vi "EFMC-3.vi"(11 "数组":u8[](array[numeric])) -> (0 "传感器信号":cluster{"陀螺温度":i16, "加计温度":i16}, 1 "组合数据来源字":T1, 2 "对准数据来源字":cluster{"位置数据":string, "姿态数据":string}, 3 "系统工作状态字":cluster{"工作状态":string, "工作模式":string})   [LabVIEW 2012]
uses:
  index-i16.vi
  XX-I16.vi
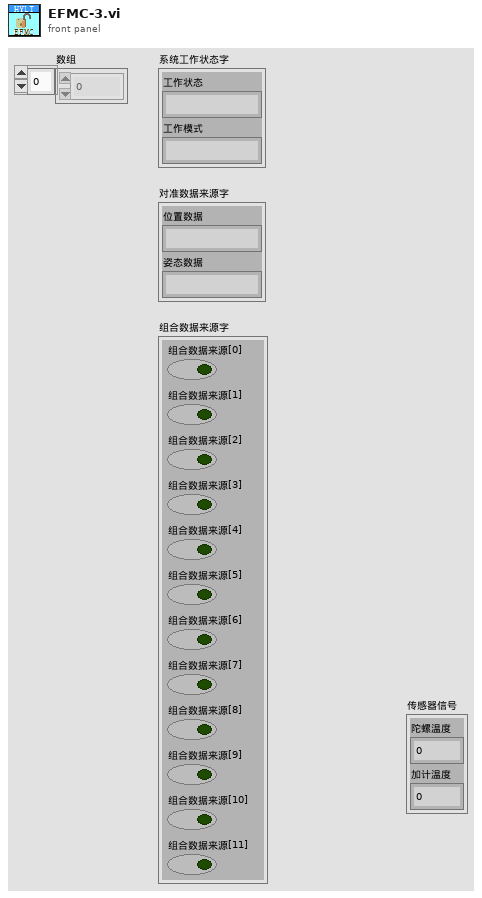
[diagram p1: front panel]
types:
  T1 = cluster{"组合数据来源[0]":bool, "组合数据来源[1]":bool, "组合数据来源[2]":bool, "组合数据来源[3]":bool, "组合数据来源[4]":bool, "组合数据来源[5]":bool, "组合数据来源[6]":bool, "组合数据来源[7]":bool, "组合数据来源[8]":bool, "组合数据来源[9]":bool, "组合数据来源[10]":bool, "组合数据来源[11]":bool}
  T2 = cluster{"GNSS1+GPS":bool, "GNSS1BD":bool, "GCSS1+GLO":bool, "GNSS3+GPS":bool, "GNSS2+GPS":bool, "GNSS2BD":bool, "GNSS2+GLO":bool, "GNSS3BD":bool, "GNSS3+GLO":bool, "大气数据":bool, "星敏1数据":bool, "星敏2数据":bool}
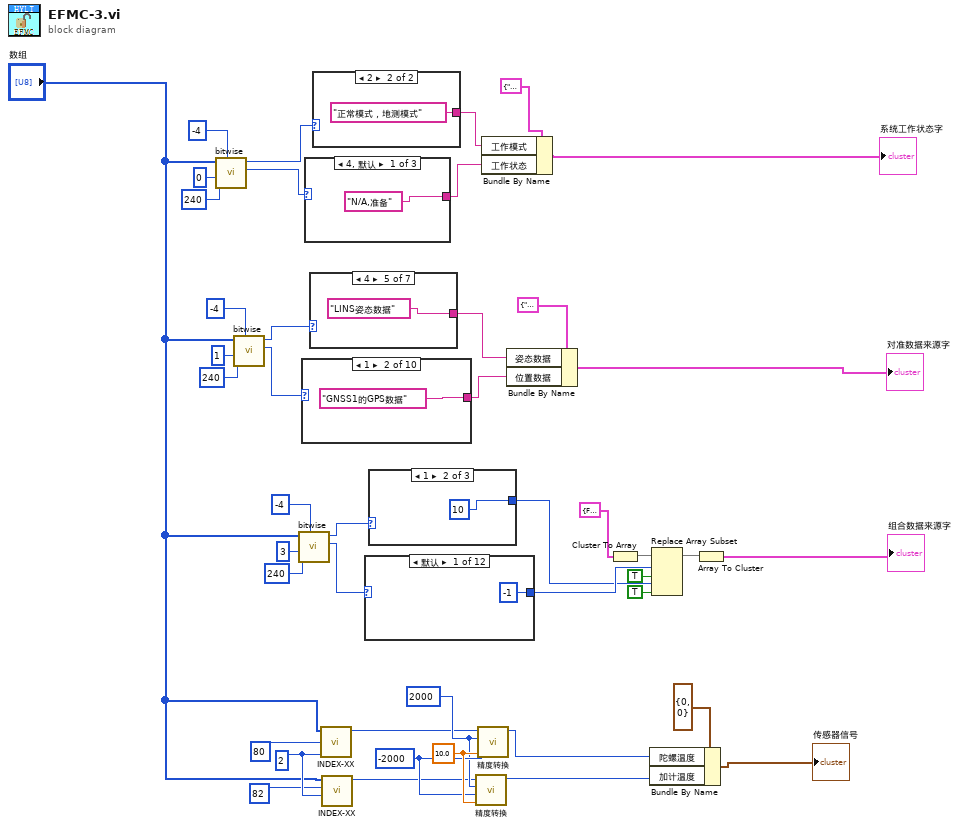
[diagram p0: block diagram]
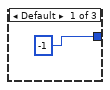
[diagram p2: hidden frame]
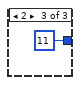
[diagram p3: hidden frame]
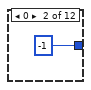
[diagram p4: hidden frame]
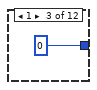
[diagram p5: hidden frame]
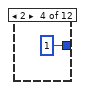
[diagram p6: hidden frame]
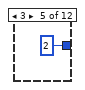
[diagram p7: hidden frame]
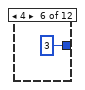
[diagram p8: hidden frame]
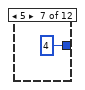
[diagram p9: hidden frame]
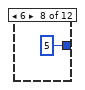
[diagram p10: hidden frame]
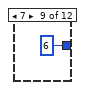
[diagram p11: hidden frame]
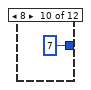
[diagram p12: hidden frame]
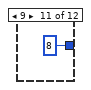
[diagram p13: hidden frame]
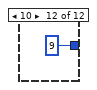
[diagram p14: hidden frame]
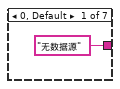
[diagram p15: hidden frame]
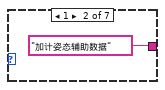
[diagram p16: hidden frame]
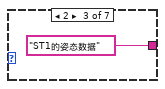
[diagram p17: hidden frame]
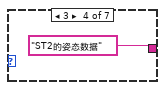
[diagram p18: hidden frame]
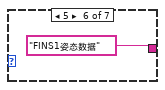
[diagram p19: hidden frame]
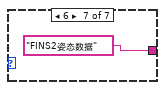
[diagram p20: hidden frame]
diagram:
  w11 = i16 -2000 ("下限")
  w10 = i16 2000 ("上限")
  w12 = 10.0 ("单位")
  w9 = 2 ("长度")
  n1 = call "bitwise.vi"("移位"=i16 -4, "置1"=u8 240, "索引"=0, "数组"="数组") -> ("y2"=w44:u8, "y1"=w43:u8)  [unwired: 6 in]
  n2 = call "bitwise.vi"("移位"=i16 -4, "置1"=u8 240, "索引"=1, "数组"="数组") -> ("y2"=w21:u8, "y1"=w22:u8)  [unwired: 6 in]
  n3 = call "bitwise.vi"("移位"=i16 -4, "置1"=u8 240, "索引"=3, "数组"="数组") -> ("y2"=w19:u8, "y1"=w20:u8)  [unwired: 6 in]
  n4 = case shown="1" w21 {
    tunnel: ["无数据源" "GNSS1的GPS数据" "GNSS2的GPS数据" "GNSS3的GPS数据" "GNSS1的BD数据" "GNSS2的BD数据" "GNSS3的BD数据" "GNSS1的GLONASS数据" "GNSS2的GLONASS数据" "GNSS3的GLONASS数据"] -> w39
    frame 0, Default {
    }
    frame 1 {
    }
    frame 2 {
    }
    frame 3 {
    }
    frame 4 {
    }
    frame 5 {
    }
    frame 6 {
    }
    frame 7 {
    }
    frame 8 {
    }
    frame 9 {
    }
  }
  n5 = case shown="4, 默认" w44 {
    tunnel: ["N/A,准备" "罗经对准，在轨对准" "导轨"] -> w42
    frame 4, Default {
    }
    frame 5 {
    }
    frame 6 {
    }
  }
  n6 = case shown="4" w22 {
    tunnel: ["无数据源" "加计姿态辅助数据" "ST1的姿态数据" "ST2的姿态数据" "LINS姿态数据" "FINS1姿态数据" "FINS2姿态数据"] -> w38
    frame 0, Default {
    }
    frame 1 {
    }
    frame 2 {
    }
    frame 3 {
    }
    frame 4 {
    }
    frame 5 {
    }
    frame 6 {
    }
  }
  n7 = case shown="2" w43 {
    tunnel: ["未知" "正常模式，地测模式"] -> w41
    frame 0, Default {
    }
    frame 2 {
    }
  }
  n8 = call-poly "INDEX-XX.vi"("长度"=w9, "索引"=80, "数组"="数组") -> ("数值输出"=w6:i16)  [unwired: 8 in]
  n9 = call-poly "INDEX-XX.vi"("长度"=w9, "索引"=82, "数组"="数组") -> ("数值输出"=w4:i16)  [unwired: 8 in]
  n10 = case shown="默认" w19 {
    tunnel: [-1 -1 0 1 2 3 4 5 6 7 8 9] -> w35
    frame Default {
    }
    frame 0 {
    }
    frame 1 {
    }
    frame 2 {
    }
    frame 3 {
    }
    frame 4 {
    }
    frame 5 {
    }
    frame 6 {
    }
    frame 7 {
    }
    frame 8 {
    }
    frame 9 {
    }
    frame 10 {
    }
  }
  n11 = case shown="1" w20 {
    tunnel: [-1 10 11] -> w32
    frame Default {
    }
    frame 1 {
    }
    frame 2 {
    }
  }
  n12 = call-poly "精度转换.vi"("单位"=w12, "下限"=w11, "上限"=w10, "数值输入"=w4) -> ("输出"=w3:i16)  [unwired: 7 in]
  n13 = call-poly "精度转换.vi"("单位"=w12, "下限"=w11, "上限"=w10, "数值输入"=w6) -> ("输出"=w5:i16)  [unwired: 7 in]
  n14 = Bundle By Name(cluster=cluster{"工作状态":string, "工作模式":string} {"工作状态"="", "工作模式"=""} ("系统状态"), "工作模式"=w41, "工作状态"=w42) -> (→"系统工作状态字":cluster{"工作状态":string, "工作模式":string})
  n15 = Bundle By Name(cluster=cluster{"位置数据":string, "姿态数据":string} {"位置数据"="", "姿态数据"=""} ("数据来源"), "姿态数据"=w38, "位置数据"=w39) -> (→"对准数据来源字":cluster{"位置数据":string, "姿态数据":string})
  n16 = Cluster To Array(cluster=T2 {"GNSS1+GPS"=FALSE, "GNSS1BD"=FALSE, "GCSS1+GLO"=FALSE, "GNSS3+GPS"=FALSE, "GNSS2+GPS"=FALSE, "GNSS2BD"=FALSE, "GNSS2+GLO"=FALSE, "GNSS3BD"=FALSE, "GNSS3+GLO"=FALSE, "大气数据"=FALSE, "星敏1数据"=FALSE, "星敏2数据"=FALSE} ("组合数据来源")) -> (array=w37:bool[])
  n17 = Bundle By Name(cluster=cluster{"陀螺温度":i16, "加计温度":i16} {"陀螺温度"=0, "加计温度"=0} ("传感器信号 3"), "陀螺温度"=w5, "加计温度"=w3) -> (→"传感器信号":cluster{"陀螺温度":i16, "加计温度":i16})
  n18 = Replace Array Subset(array=w37, new element #1=TRUE ("新元素/子数组"), index #1=w35, new element #2=TRUE ("新元素/子数组"), index #2=w32) -> (w34:bool[])
  n19 = Array To Cluster(array=w34) -> (cluster=→"组合数据来源字":T1)
